vi "MStarDailyTooling.vi"() -> ()   [LabVIEW 2012]
uses:
  <vilib>/Utility/NIReport.llb/NI_report.lvclass
  <vilib>/addons/database/Connection.llb/DB Tools Open Connec (Path).vi
  <vilib>/addons/database/Connection.llb/Conn Execute.vi
  <vilib>/addons/database/Recordset.llb/Rec Fetch Recordset Data (R).vi
  <vilib>/addons/database/Recordset.llb/Rec Destroy - Connection.vi
  <vilib>/Utility/NIReport.llb/Append Text Table to Report (wrap).vi
  <vilib>/addons/database/_DB Variant To Data/Database Variant To Data.xnode
  <vilib>/addons/database/NI_Database_API.lvlib
  <vilib>/Utility/NIReport.llb/Excel/NI_Excel.lvclass
  <vilib>/Utility/SMTP/NI_SMTPEmail.lvlib
panel:
  in  "Report Template":path=path "O:/Monitor/Report/MSTTooling.xls"
  out "error out 2":errorcluster
  in  "Table Control":string[][](table)
  out "error out 3":errorcluster
  out "appended array":string[](array[string])
  out "recordset data":variant[][](array[variant])
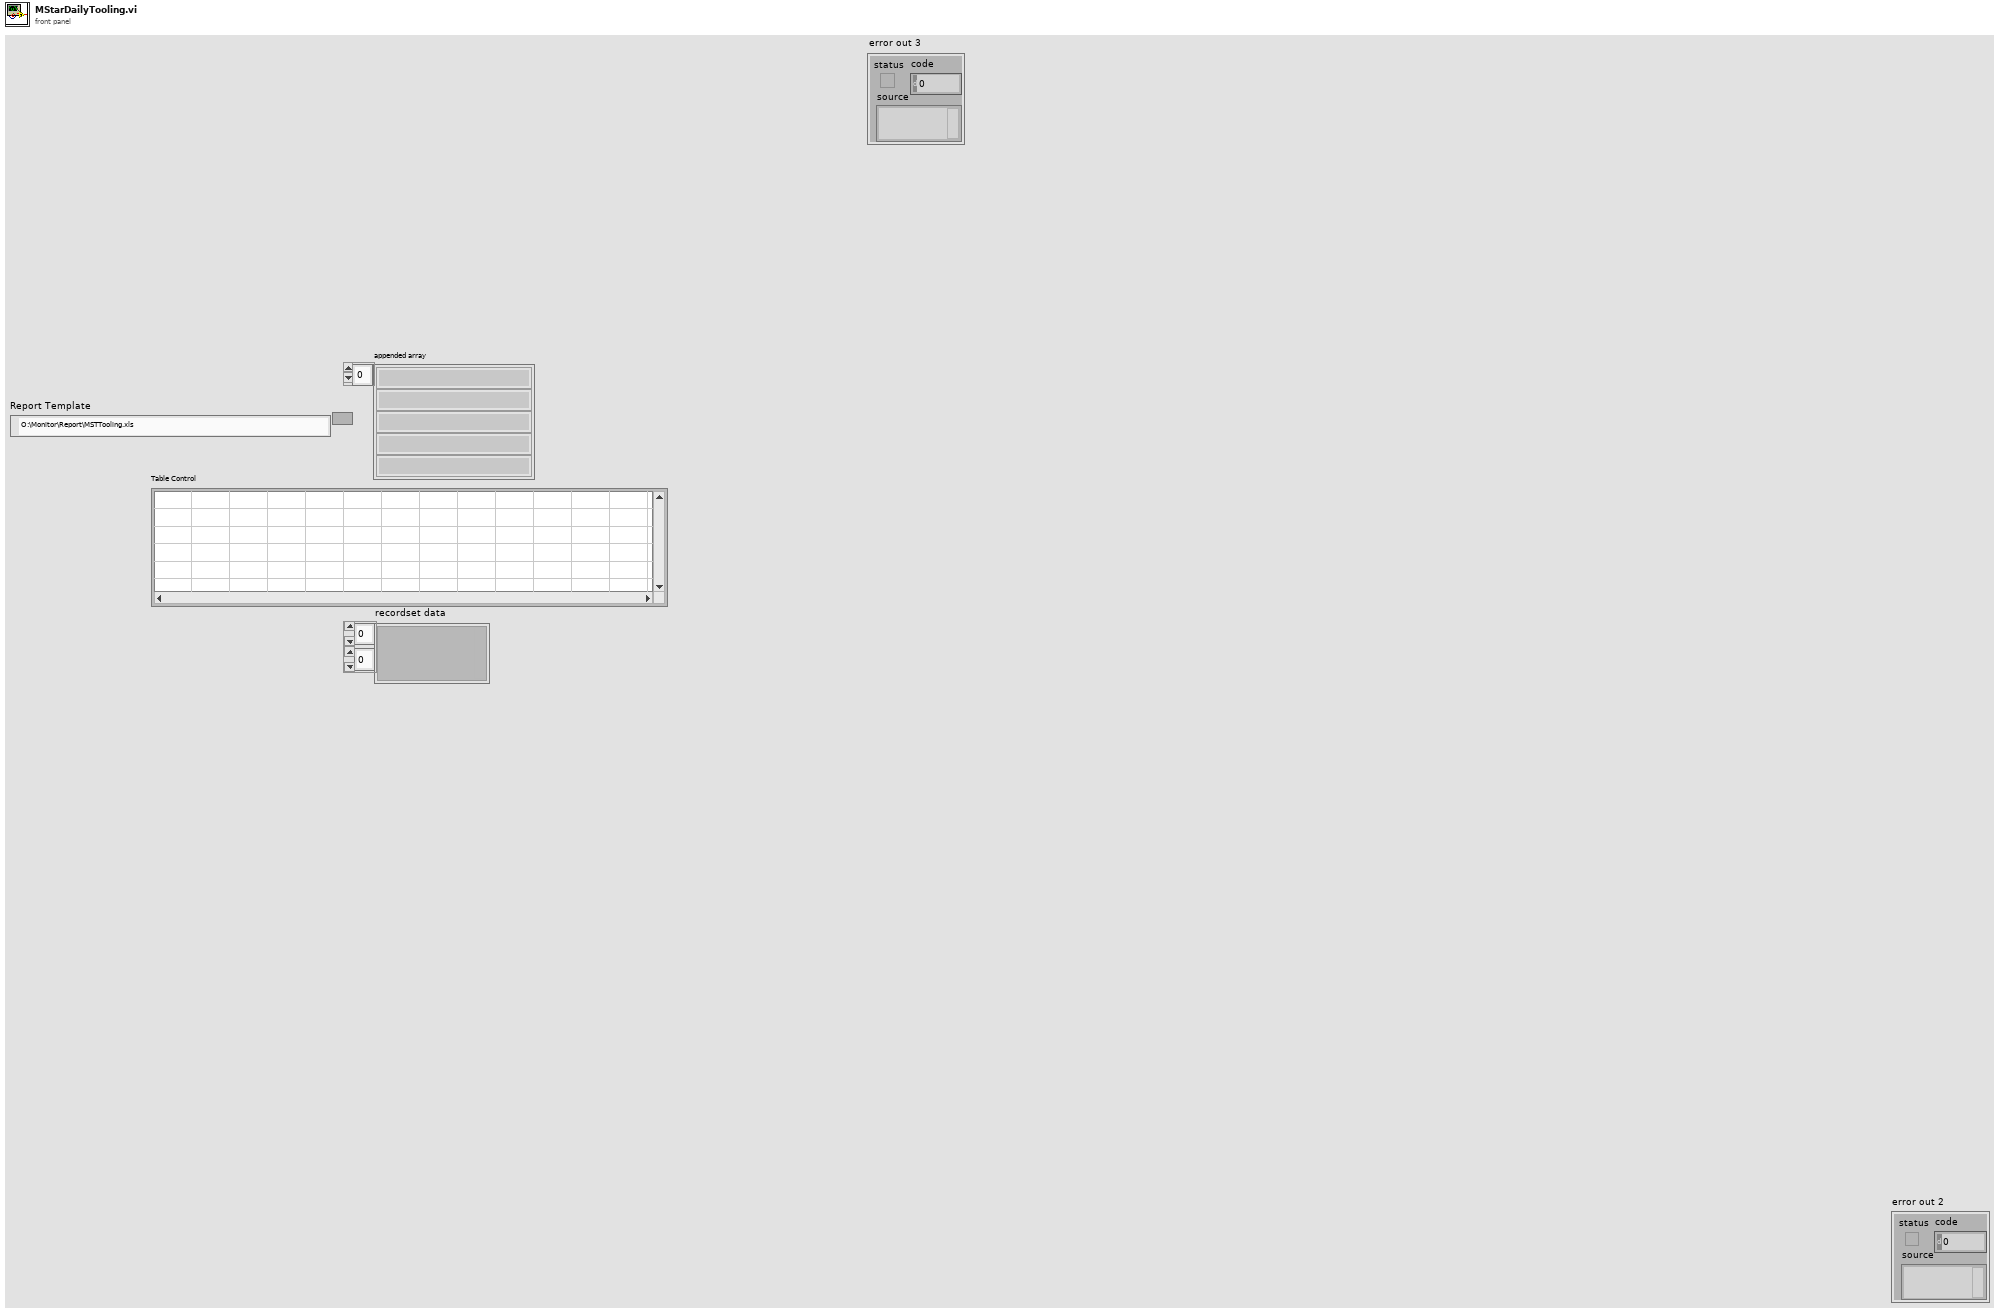
[diagram p1: front panel]
types:
  T1 = typedef "NI_Database_API.lvlib/Conn ObjectReference.ctl" = refnum<k1>
  T2 = typedef "NI_Database_API.lvlib/Rec ObjectReference.ctl" = refnum<k1>
  T3 = enum16{"Standard Report", "HTML", "Word", "Excel"}
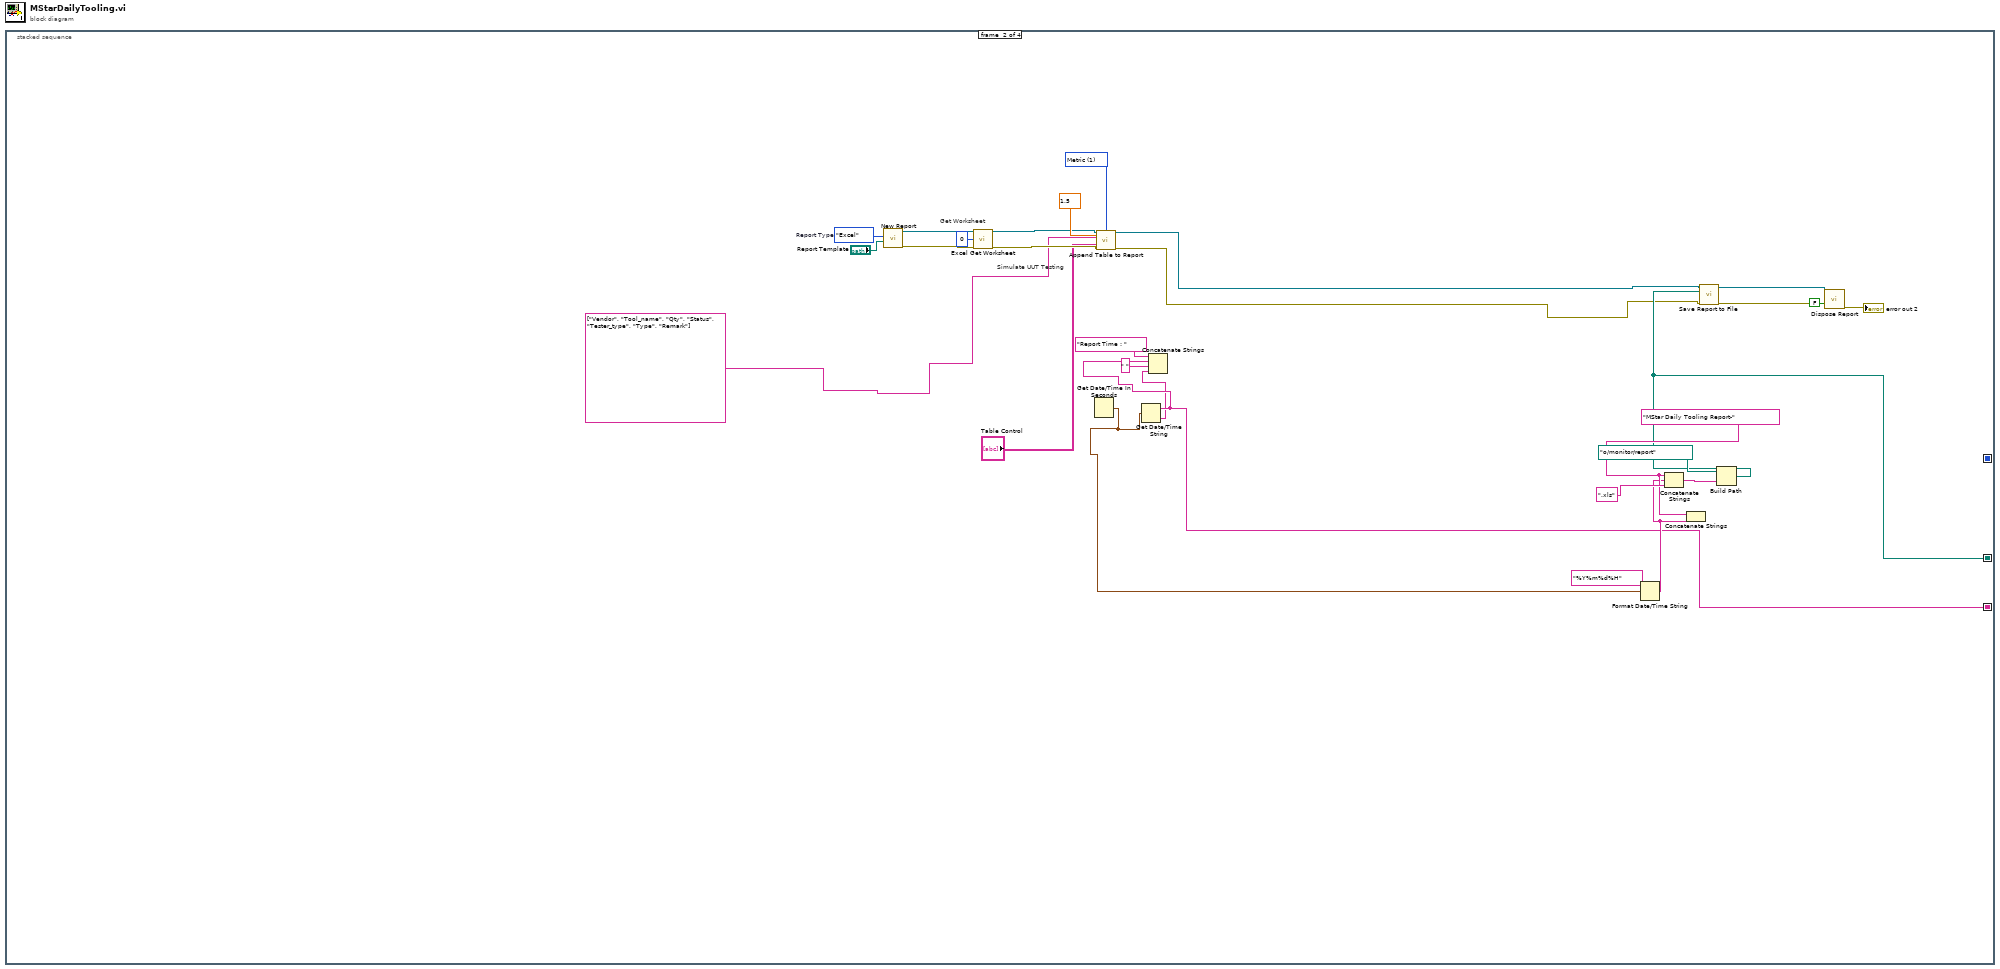
[diagram p0: block diagram]
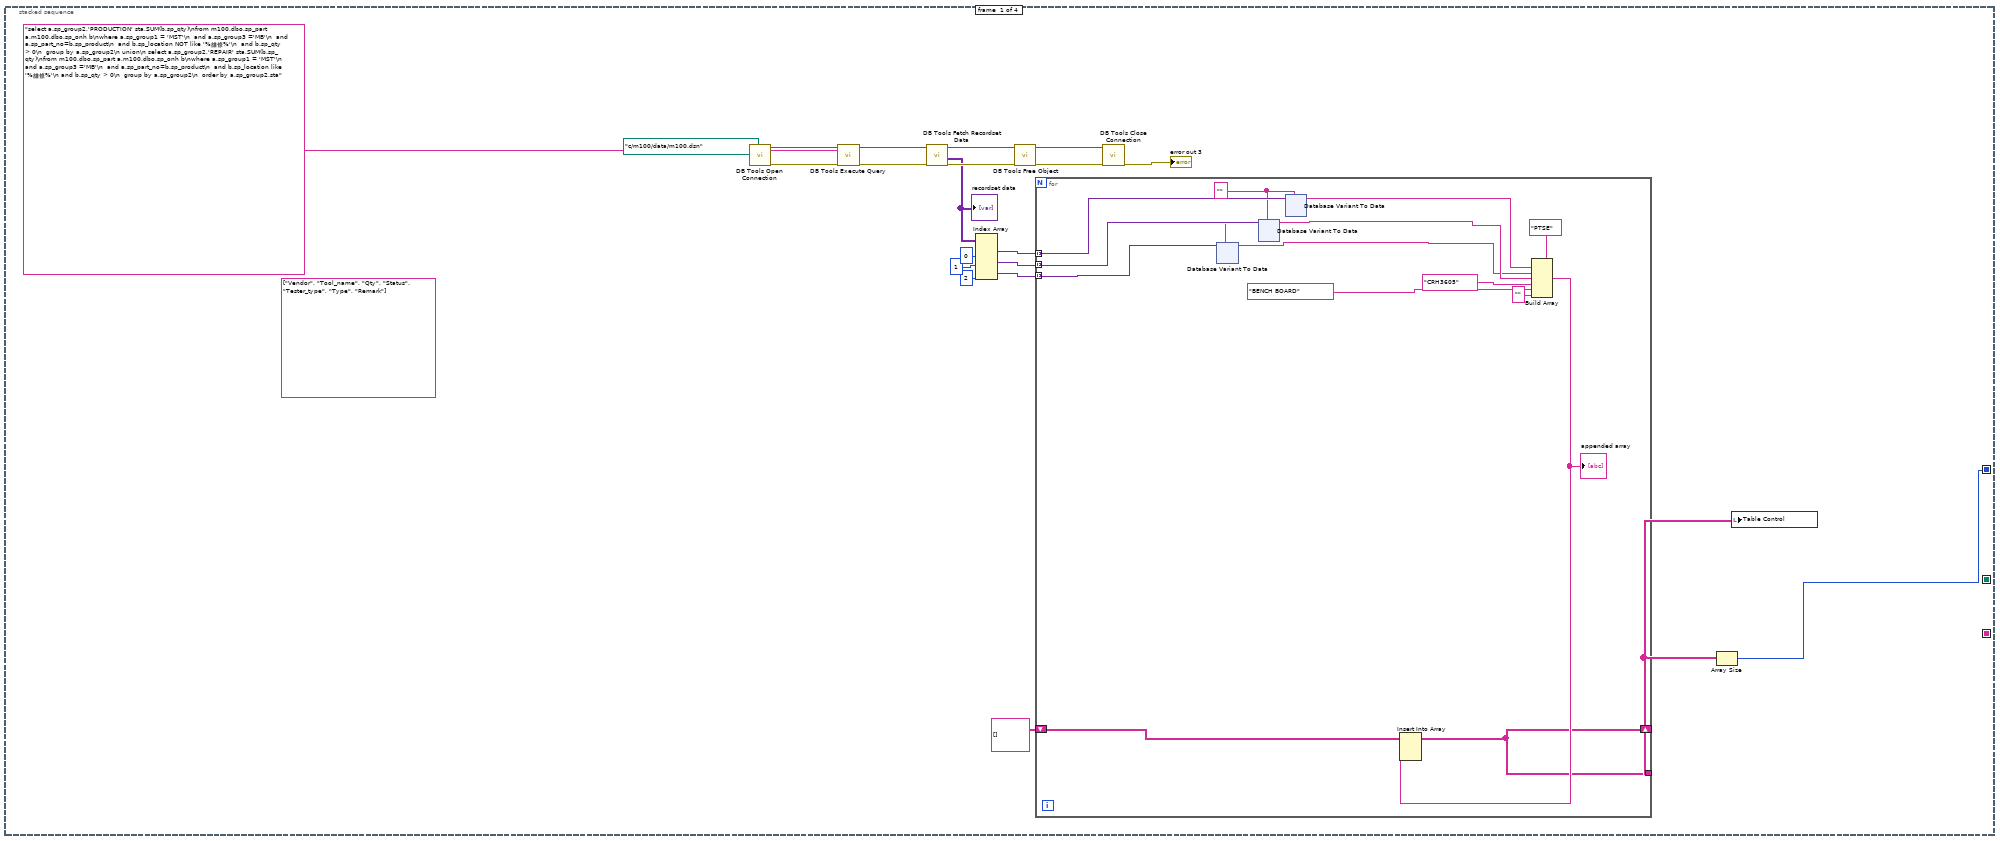
[diagram p2: hidden frame]
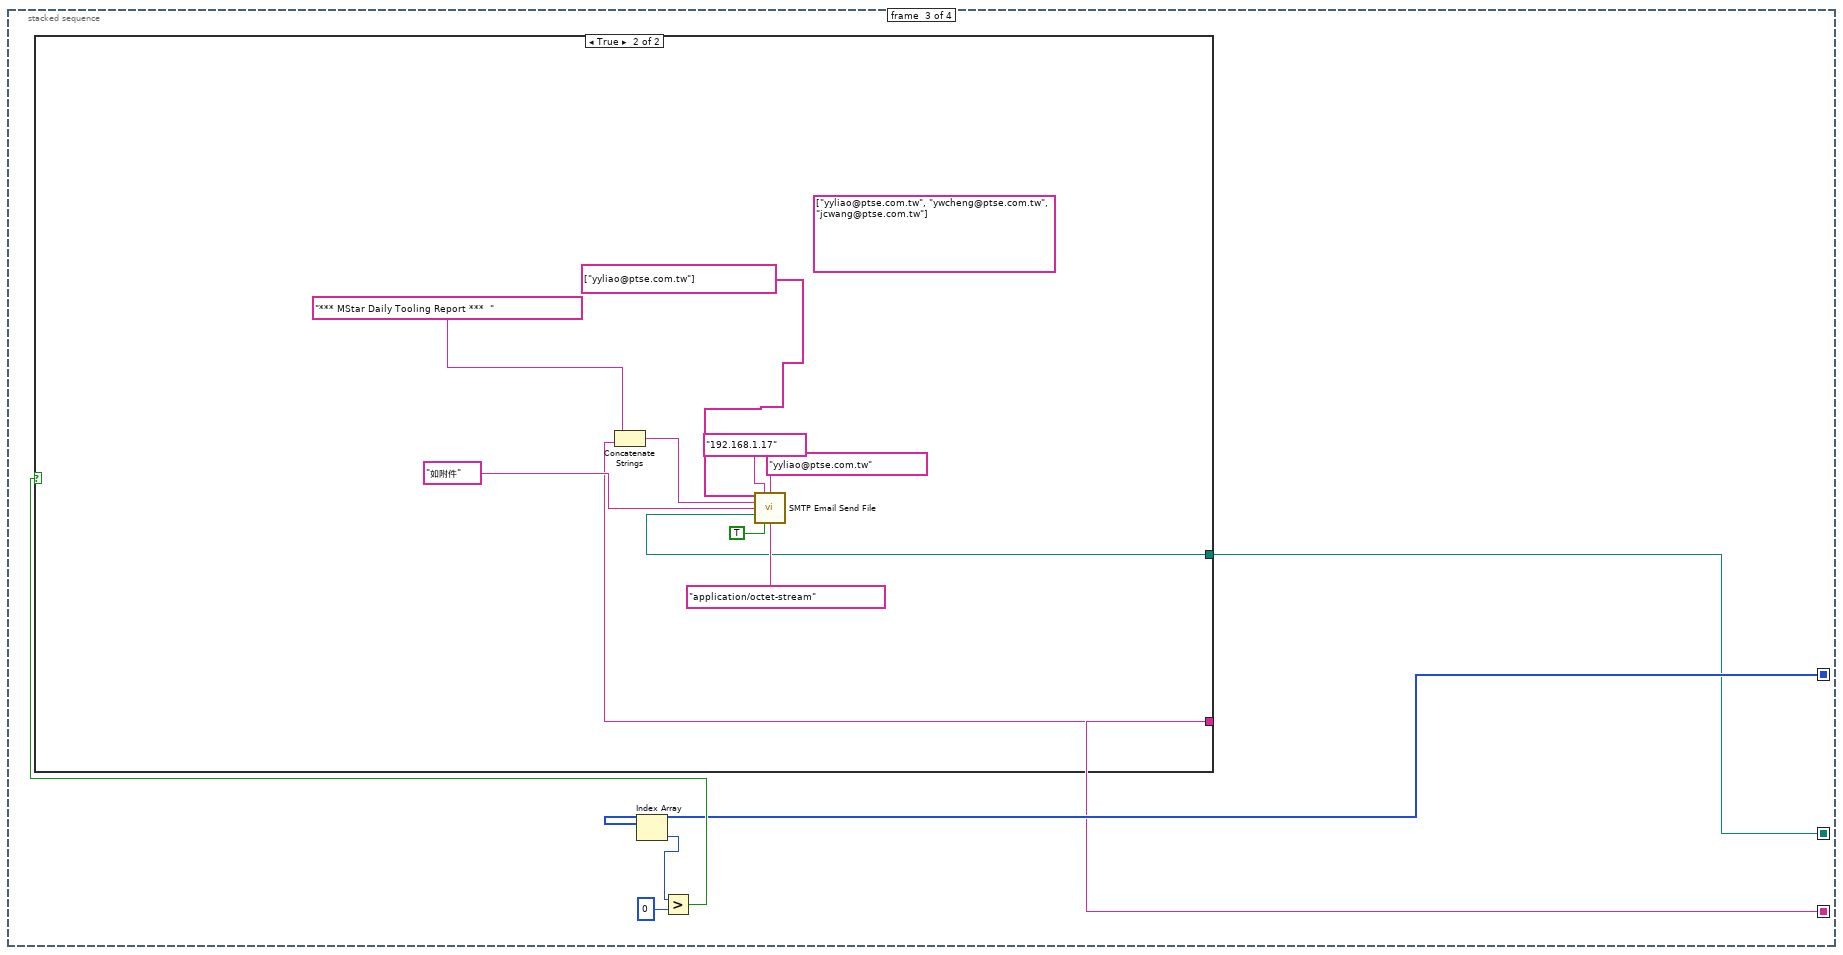
[diagram p3: hidden frame]
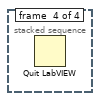
[diagram p5: hidden frame]
diagram:
  n1 = stacked-sequence {
    seq-local: [w1 _ _ _] -> [_ _ w163 _]
    seq-local: [_ w140 _ _] -> [_ _ w162 _]
    seq-local: [_ w137 _ _] -> [_ _ w161 _]
    frame #0 {
      (unwired) string[] ["Vendor", "Tool_name", "Qty", "Status", "Tester_type", "Type", "Remark"] ("row headers")
      n2 = call-poly <vilib>:"DB Tools Open Connection.vi"("connection information"=path "c:/m100/data/m100.dsn") -> ("error out"=w16:errorcluster, "connection reference"=w20:T1)  [unwired: 7 in]
      n3 = call-poly <vilib>:"DB Tools Execute Query.vi"("error in (no error)"=w16, "SQL query"="select a.sp_group2,'PRODUCTION' sta,SUM(b.sp_qty)\nfrom m100.dbo.sp_part a,m100.dbo.sp_onh b\nwhere a.sp_group1 = 'MST'\n  and a.sp_group3 ='MB'\n  and a.sp_part_no=b.sp_product\n  and b.sp_location NOT like '%維修%'\n  and b.sp_qty > 0\n  group by a.sp_group2\n union\n select a.sp_group2,'REPAIR' sta,SUM(b.sp_qty)\nfrom m100.dbo.sp_part a,m100.dbo.sp_onh b\nwhere a.sp_group1 = 'MST'\n  and a.sp_group3 ='MB'\n  and a.sp_part_no=b.sp_product\n  and b.sp_location like '%維修%'\n and b.sp_qty > 0\n  group by a.sp_group2\n  order by a.sp_group2,sta", "connection reference"=w20) -> ("error out"=w15:errorcluster, "recordset reference"=w19:T2)  [unwired: 5 in]
      n4 = call-poly <vilib>:"DB Tools Fetch Recordset Data.vi"("error in (no error)"=w15, "recordset reference"=w19) -> ("error out"=w14:errorcluster, "recordset data"=w4:variant[][], "recordset reference out"=w18:T2)  [unwired: 3 in]
      "recordset data" <- w4
      n5 = Index Array(array=w4, index (col) #1=0 ("disabled index (col)"), index (col) #2=1 ("index (col)"), index (col) #3=2 ("index (col)")) -> (element #1=w8:variant[], element #2=w7:variant[], element #3=w6:variant[])  [unwired: 3 in]
      n6 = call-poly <vilib>:"DB Tools Free Object.vi"("error in (no error)"=w14, "recordset reference"=w18) -> ("error out"=w13:errorcluster, "connection reference"=w17:T1)  [unwired: 8 in]
      n7 = for {
        tunnel: w8 -> [w35] mode=indexing
        tunnel: w7 -> [w34] mode=indexing
        tunnel: w6 -> [w33] mode=indexing
        tunnel: [w31] -> w2
        shift-right: [w31] -> _
        shift-left: string[][] [] -> [w30]
        w28 = ""
        n8 = xnode "Database Variant To Data"("database variant"=w33, "type"=w28) -> ("data"=w25:string)  [unwired: 1 in, 1 out]
        n9 = xnode "Database Variant To Data"("database variant"=w34, "type"=w28) -> ("data"=w29:string)  [unwired: 1 in, 1 out]
        n10 = xnode "Database Variant To Data"("database variant"=w35, "type"=w28) -> ("data"=w26:string)  [unwired: 1 in, 1 out]
        n11 = Build Array("PTSE", w26, w25, w29, "CRH3605" ("element"), "BENCH BOARD" ("element"), "" ("element")) -> (w32:string[])
        "appended array" <- w32
        n12 = Insert Into Array(array=w30, new element=w32) -> (w31:string[][])  [unwired: 2 in]
      }
      n13 = call <vilib>:"DB Tools Close Connection.vi"("error in (no error)"=w13, "connection reference"=w17) -> ("error out"=→"error out 3":errorcluster)  [unwired: 5 in]
      n14 = Array Size(array=w2) -> (size(s)=w1:i32[])
      n15 = local write "Table Control"(w2) -> ()
    }
    frame #1 {
      w144 = u16 1 items=["US", "Metric", "Default"] ("measurement system")
      w145 = "MStar Daily Tooling Report-"
      w160 = T3."Excel"  # Report Type
      # "Simulate UUT Testing"
      # "Get Worksheet"
      n16 = call <vilib>:"New Report.vi"("report type"=w160, "template (empty)"="Report Template") -> ("report out"=w157:refnum<class "NI_report.lvclass">, "error out"=w156:errorcluster)  [unwired: 12 in]
      n17 = call <vilib>:"Excel Get Worksheet.vi"("report in"=w157, "worksheet index (0)"=0, "error in (no error)"=w156) -> ("report out"=w150:refnum<class "NI_report.lvclass">, "error out"=w149:errorcluster)  [unwired: 11 in]
      n18 = Get Date/Time In Seconds() -> (seconds since 1Jan1904=w135:timestamp)
      n19 = call-poly <vilib>:"Append Table to Report.vi"("report in"=w150, "column width (1)"=1.5, "measurement system"=w144, "column headers"=string[] ["Vendor", "Tool_name", "Qty", "Status", "Tester_type", "Type", "Remark"] ("row headers"), "text data"="Table Control", "error in (no error)"=w149) -> ("report out"=w134:refnum<class "NI_report.lvclass">, "error out"=w133:errorcluster)  [unwired: 6 in, 2 out]
      n20 = Get Date/Time String(seconds (now)=w135) -> (date string=w137:string, time string=w136:string)  [unwired: 2 in]
      n21 = Concatenate Strings("Report Time : " ("string"), w137, " " ("string"), w136) -> ()  [unwired: 1 out]
      n22 = Format Date/Time String(time format string (%c)="%Y%m%d%H", seconds (now)=w135) -> (date/time string=w142:string)  [unwired: 1 in]
      n23 = Concatenate Strings(w145, w142, ".xls" ("string")) -> (w146:string)
      n24 = Concatenate Strings(w145, w142) -> ()  [unwired: 1 out]
      n25 = Build Path(base path=path "o:/monitor/report", name or relative path=w146) -> (appended path=w140:path)
      n26 = call-dynamic "Save Report to File.vi"("report in"=w134, "report file path"=w140, "error in (no error)"=w133) -> ("report out"=w152:refnum<class "NI_report.lvclass">, "error out"=w151:errorcluster)  [unwired: 11 in]
      n27 = call-dynamic "Dispose Report.vi"("report in"=w152, "save changes? (F)"=FALSE, "error in (no error)"=w151) -> ("error out"=→"error out 2":errorcluster)  [unwired: 12 in]
    }
    frame #2 {
      n28 = Index Array(array=w163) -> (element=w166:i32)  [unwired: 1 in]
      n29 = Greater?(x=w166, y=0) -> (0:w164:bool)
      n30 = case shown="True" w164 {
        tunnel: w162 -> [_ w171]
        tunnel: w161 -> [_ w168]
        frame False {
        }
        frame True {
          (unwired) string[] ["yyliao@ptse.com.tw", "ywcheng@ptse.com.tw", "jcwang@ptse.com.tw"] ("recipients")
          n31 = Concatenate Strings("*** MStar Daily Tooling Report ***  " ("subject ([No Subject])"), w168) -> (w169:string)
          n32 = call <vilib>:"SMTP Email Send File.vi"("recipients"=string[] ["yyliao@ptse.com.tw"], "mail server"="192.168.1.17", "return address"="yyliao@ptse.com.tw", "subject ([No Subject])"=w169, "message"="如附件", "file path"=w171, "binary? (F)"=TRUE, "MIME content-type (application/octet-stream)"="application/octet-stream") -> ()  [unwired: 6 in, 2 out]
        }
      }
    }
    frame #3 {
      n33 = Quit LabVIEW() -> ()  [unwired: 1 in]
    }
  }
